vi "Set Default DAQ Port1 State.vi"(0 "TSM Context":T1) -> (15 "error out":errorcluster)   [LabVIEW 2019]
uses:
  <vilib>/NI_TestStand_SemiconductorModule/NI_TestStand_Semiconductor_Module.lvlibp/PinMap/General/SemiconductorModuleContext.ctl
  TSM Context Data Access/TSM Context Data Access.lvclass/TSM Context Data Access.ctl
  TSM Context Data Access/Public/Properties/DAQ Port1 State - Write.vi
  TSM Context Data Access/Public/Properties/DAQ Port1 Pins - Write.vi
  <vilib>/NI_TestStand_SemiconductorModule/NI_TestStand_Semiconductor_Module.lvlibp/PinMap/Site and Global Data/SetGlobalData.vi
  TSM Context Data Access/TSM Context Data Access.lvclass
  <vilib>/NI_TestStand_SemiconductorModule/NI_TestStand_Semiconductor_Module.lvlibp
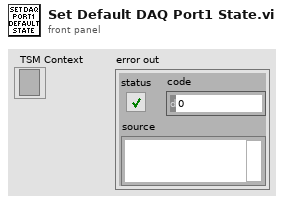
[diagram p1: front panel]
types:
  T1 = typedef "NI_TestStand_Semiconductor_Module.lvlibp/SemiconductorModuleContext.ctl" = refnum<k7>
  T2 = typedef "TSM DAQmx.ctl" = cluster{"Pin Query Context":refnum<class "MultiplePinSingleSessionQueryContext.lvclass">, "SSC":T3, "Site Numbers":i32[]}
  T3 = typedef "SSC DAQmx.ctl" = cluster{"DAQmx Task ":refnum<k21>, "Channels":string, "Channel Lists":string}
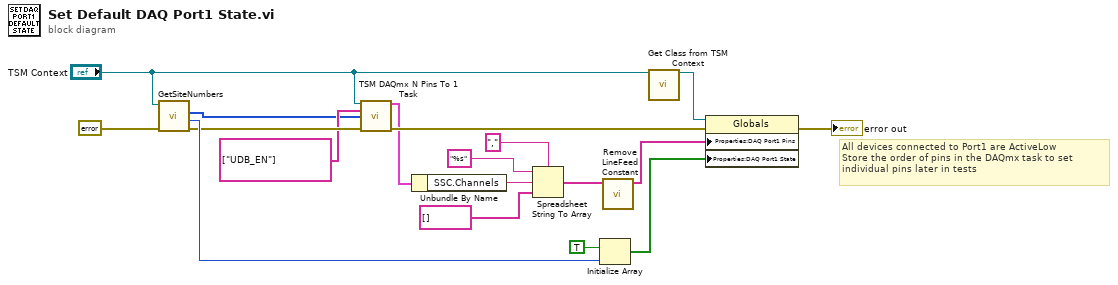
[diagram p0: block diagram]
diagram:
  # "All devices connected to Port1 are ActiveLow\nStore the order of pins in the DAQmx task to set individual pins later in tests"
  n1 = call <vilib>:"GetSiteNumbers.vi"("error in (no error)"=errorcluster {"status"=FALSE, "code"=0, "source"=""} ("error in"), "Semiconductor Module Context"="TSM Context") -> ("error out"=w13:errorcluster, "Number Of Sites"=w16:i32, "Site Numbers"=w9:i32[])  [unwired: 6 in, 1 out]
  n2 = call "TSM DAQmx N Pins To 1 Task.vi"("TSM context"="TSM Context", "Pins"=string[] ["UDB_EN"], "Site Numbers"=w9, "error in"=w13) -> ("DAQ TSM Out"=w11:T2, "error out"=w12:errorcluster)  [unwired: 10 in]
  n3 = Unbundle By Name(w11) -> ("SSC.Channels"=w8:string)
  n4 = Spreadsheet String To Array(delimiter (Tab)=",", format string="%s", spreadsheet string=w8, array type (2D Dbl)=string[] []) -> (array=w2:string[])
  n5 = Initialize Array(TRUE, w16) -> (w4:bool[])
  n6 = call "Remove LineFeed Constant.vi"("1D String Array in"=w2) -> ("1D String Array out"=w1:string[])  [unwired: 10 in]
  n7 = call "Get Class from TSM Context.vi"("TSM Context"="TSM Context") -> ("Global Memory Class"=w18:refnum<class "TSM Context Data Access.lvclass">)  [unwired: 14 in]
  n8 = property class="Globals"(reference=w18, error in=w12, "Properties:DAQ Port1 Pins"=w1, "Properties:DAQ Port1 State"=w4) -> (error out=→"error out":errorcluster)  [unwired: 1 out]
